vi "Send_SET_1BIT.vi"(8 "error in (no error)":errorcluster, 9 "Encender?":bool, 10 "Channel":u8, 11 "Simulated uC in":refnum<class "Simulated uC.lvclass">) -> (0 "error out":errorcluster, 2 "buffer":string, 3 "Simulated uC out":refnum<class "Simulated uC.lvclass">)   [LabVIEW 2019, in "Simulated uC.lvclass"]
uses:
  Simulated uC.lvclass
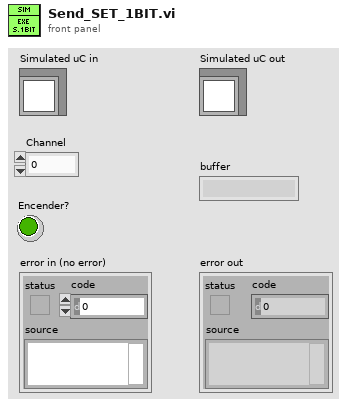
[diagram p1: front panel]
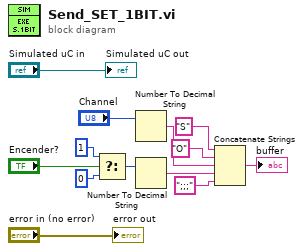
[diagram p0: block diagram]
diagram:
  n1 = Select(t=u8 1 ("Channel"), s="Encender?", f=u8 0 ("Channel")) -> (s? t:f=w4:u8)
  n2 = Number To Decimal String(number="Channel") -> (decimal integer string=w8:string)  [unwired: 1 in]
  n3 = Number To Decimal String(number=w4) -> (decimal integer string=w3:string)  [unwired: 1 in]
  n4 = Concatenate Strings("S" ("string"), "O" ("string"), w8, w3, ";;;" ("string")) -> (→"buffer":string)
  "error out" <- "error in (no error)"
  "Simulated uC out" <- "Simulated uC in"
